vi "Handle getAll.vi"(8 "error in (no error)":errorcluster, 11 "Instrument.AFM_DLog in":refnum<class "Instrument.AFM_DLog.lvclass">) -> (0 "error out":errorcluster, 2 "getAll":variant, 3 "Instrument.AFM_DLog out":refnum<class "Instrument.AFM_DLog.lvclass">)   [LabVIEW 2019, in "Instrument.AFM_DLog.lvclass"]
uses:
  Instrument.AFM_DLog.lvclass
  Instrument.AFM_DLog.lvclass/Instrument.AFM_DLog.ctl
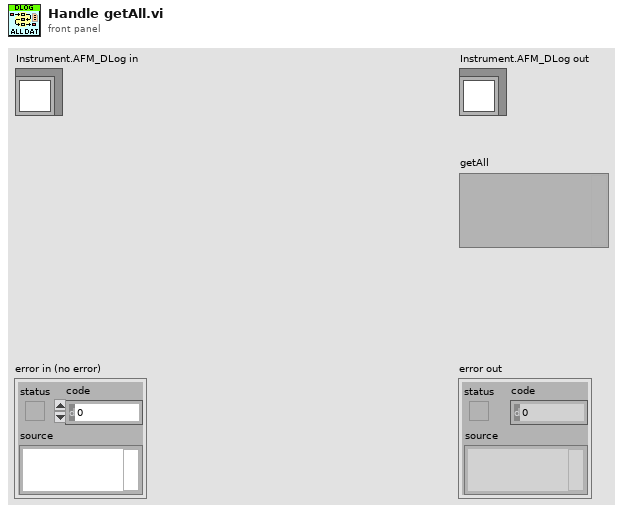
[diagram p1: front panel]
types:
  T1 = typedef "Instrument.AFM_DLog.lvclass/Instrument.AFM_DLog.getAll--Cluster.ctl" = cluster{"Levy 1":dbl, "Logger SMO":dbl, "SMO Boolean":bool, "SMO String":string}
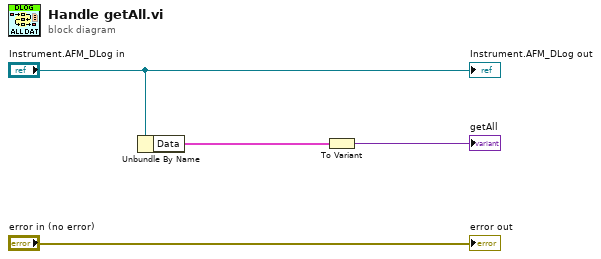
[diagram p0: block diagram]
diagram:
  n1 = Unbundle By Name("Instrument.AFM_DLog in") -> ("Data"=w1:T1)
  n2 = To Variant(anything=w1) -> (Variant=→"getAll":variant)
  "error out" <- "error in (no error)"
  "Instrument.AFM_DLog out" <- "Instrument.AFM_DLog in"
